vi "programa1.vi"() -> ()   [LabVIEW 2011]
panel:
  out "Multiplicacion":dbl
  out "Division":dbl
  out "Resta":dbl
  out "Suma":dbl
  in  "Numero2":dbl
  in  "Numero1":dbl
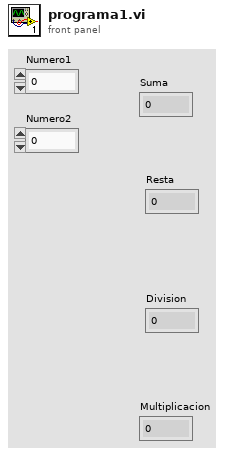
[diagram p1: front panel]
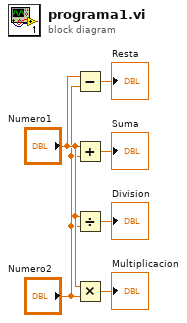
[diagram p0: block diagram]
diagram:
  n1 = Subtract(x="Numero1", y="Numero2") -> (x-y=→"Resta":dbl)
  n2 = Add(x="Numero1", y="Numero2") -> (x+y=→"Suma":dbl)
  n3 = Divide(x="Numero1", y="Numero2") -> (x/y=→"Division":dbl)
  n4 = Multiply(x="Numero1", y="Numero2") -> (x*y=→"Multiplicacion":dbl)
